vi "ClientSide.vi"() -> ()   [LabVIEW 2019]
panel:
  out "length":i32
  out "Msg":string
  out "Full Name":string
  out "Your Age":dbl
  in  "type":T1
  in  "Stop Client side":bool
  out "error out":errorcluster
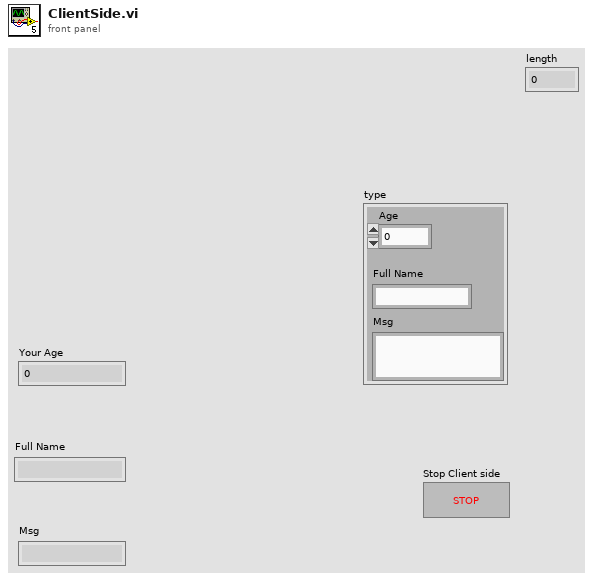
[diagram p1: front panel]
types:
  T1 = cluster{"Age":dbl, "Msg":string, "Full Name ":string}
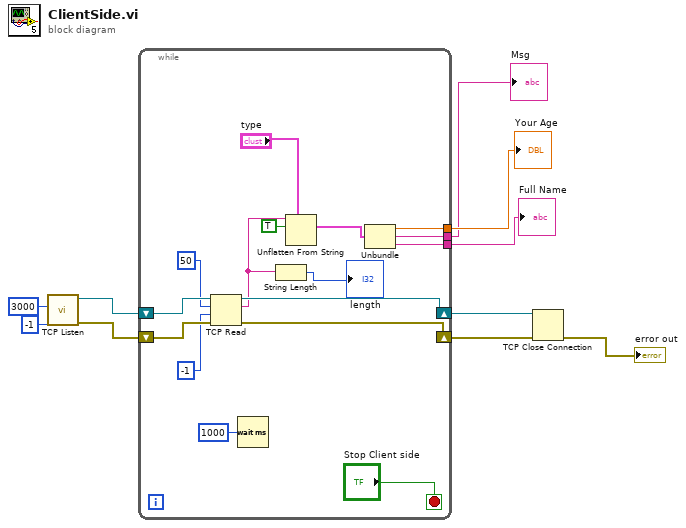
[diagram p0: block diagram]
diagram:
  n1 = call <vilib>:"TCP Listen.vi"("timeout ms (wait forever: -1)"=-1, "port"=u16 3000) -> ("error out"=w8:errorcluster, "connection ID"=w10:refnum<k5>)  [unwired: 5 in, 3 out]
  n2 = while {
    shift-right: [w25] -> w9
    shift-left: w10 -> [w26]
    shift-right: [w23] -> w7
    shift-left: w8 -> [w24]
    tunnel: [w16] -> w3
    tunnel: [w15] -> w2
    tunnel: [w14] -> w1
    stop <- "Stop Client side" stop-if-true
    n3 = TCP Read(connection ID=w26, bytes to read=50, error in (no error)=w24, 9:-1 ("timeout ms (25000)")) -> (connection ID out=w25:refnum<k5>, data out=w11:string, error out=w23:errorcluster)  [unwired: 1 in]
    n4 = Wait (ms)(milliseconds to wait=u32 1000) -> ()  [unwired: 1 out]
    n5 = String Length(string=w11) -> (length=→"length":i32)
    n6 = Unflatten From String(type="type", binary string=w11, data includes array or string size? (T)=TRUE) -> (value=w17:T1)  [unwired: 2 in, 2 out]
    n7 = Unbundle(w17) -> ("Age"=w16:dbl, "Msg"=w15:string, "Full Name"=w14:string)
  }
  "Your Age" <- w3
  "Full Name" <- w1
  "Msg" <- w2
  n8 = TCP Close Connection(connection ID=w9, error in (no error)=w7) -> (error out=→"error out":errorcluster)  [unwired: 1 in, 1 out]
